vi "01AMT800_AnalyzeReceive.vi"(8 "error in (no error)":errorcluster, 10 "String":string, 11 "Enum":enum16{"Initialize", "Analyze"}(ring)) -> (0 "error out":errorcluster, 3 "Data":T1)   [LabVIEW 2015]
uses:
  <vilib>/regexp/Match Regular Expression.xnode
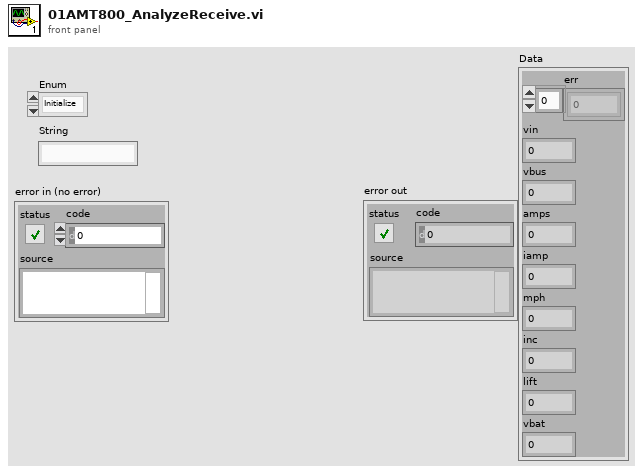
[diagram p1: front panel]
types:
  T1 = cluster{"err":i32[], "vin":i32, "vbus":i32, "amps":i32, "iamp":i32, "mph":i32, "inc":i32, "lift":i32, "vbat":i32}
  T2 = enum16{"Initialize", "Next", "Send RSET", "Set MPH", "Set INC", "Part to 0"}
  T3 = enum16{"Initialize", "FootReceive", "FootDisplay"}
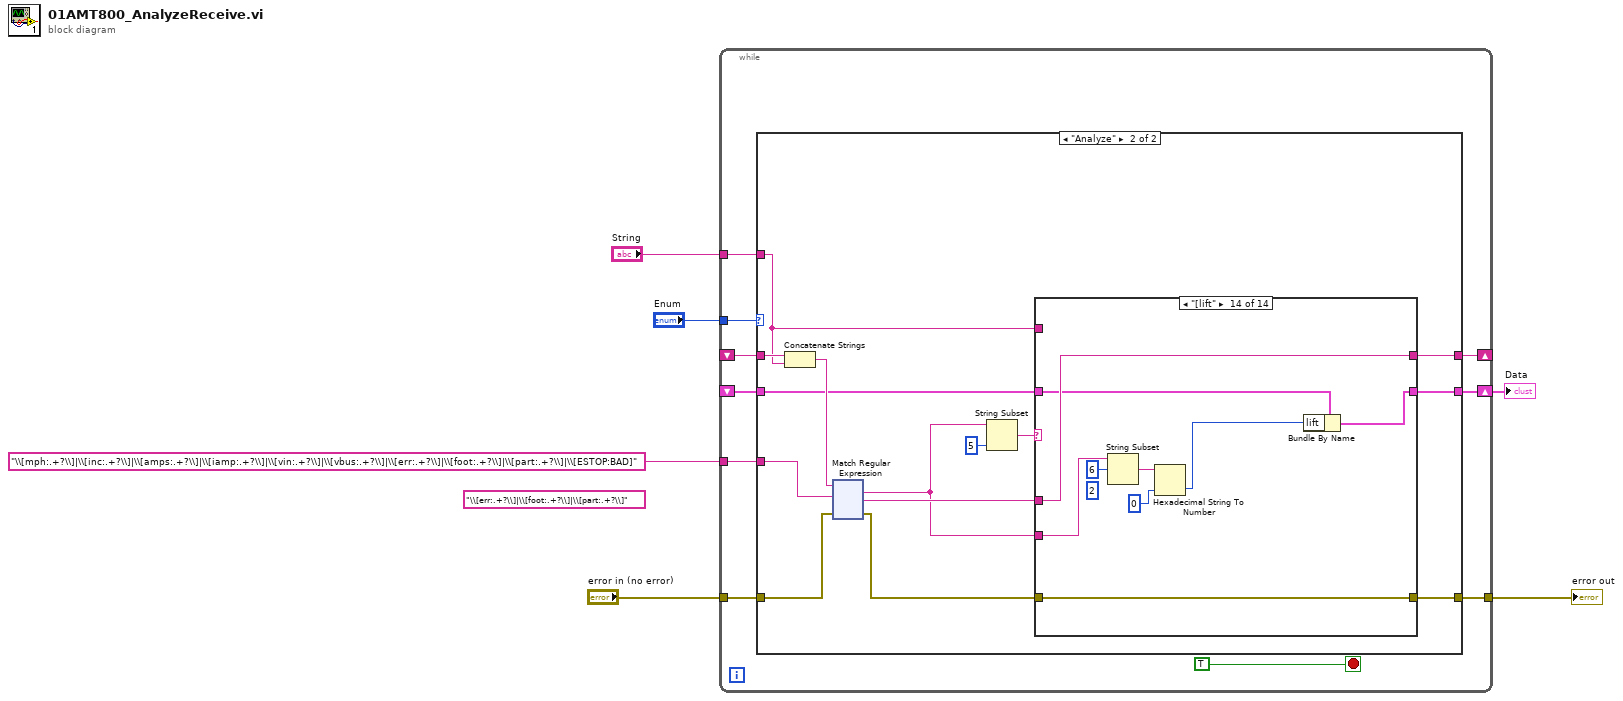
[diagram p0: block diagram]
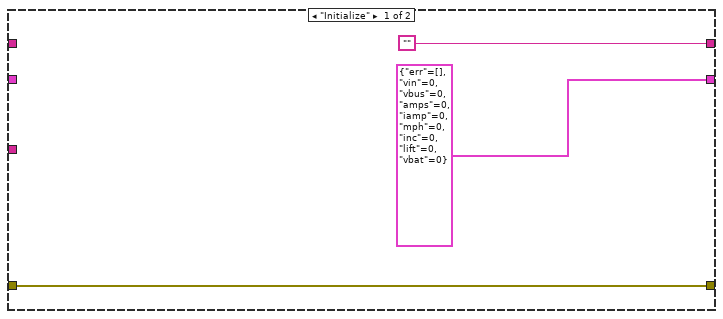
[diagram p2: hidden frame]
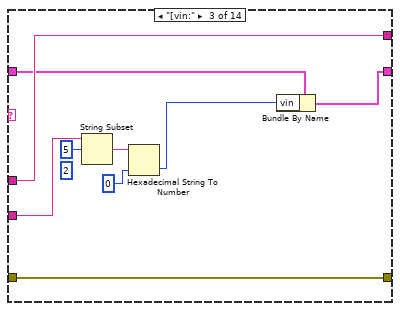
[diagram p5: hidden frame]
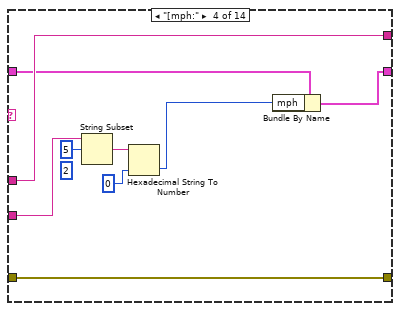
[diagram p6: hidden frame]
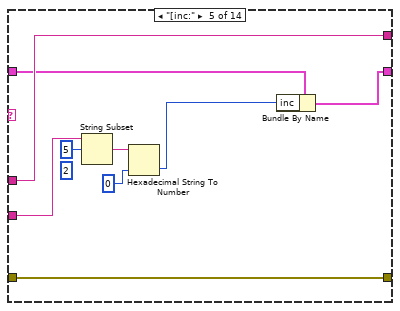
[diagram p7: hidden frame]
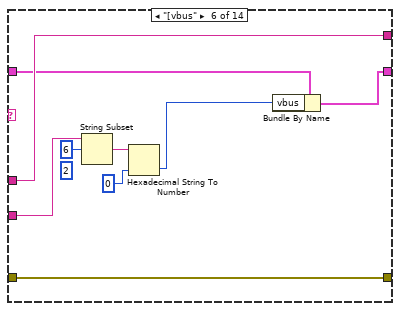
[diagram p8: hidden frame]
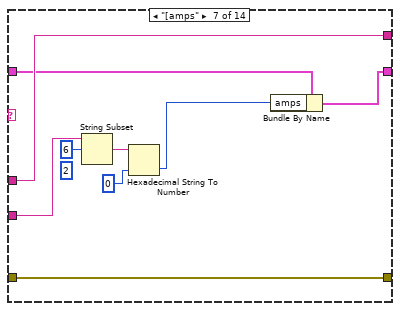
[diagram p9: hidden frame]
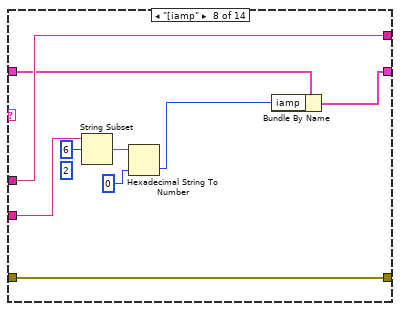
[diagram p10: hidden frame]
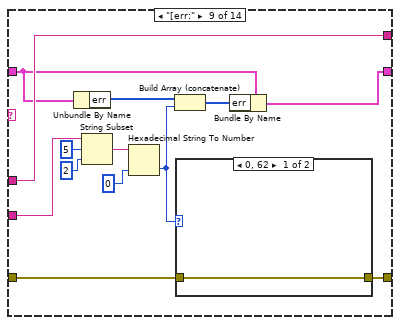
[diagram p11: hidden frame]
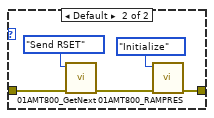
[diagram p12: hidden frame]
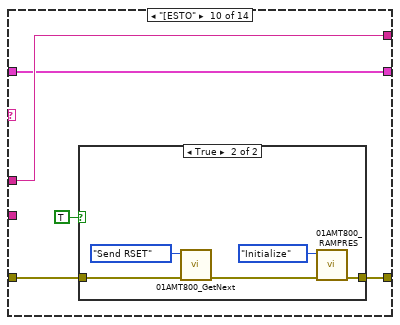
[diagram p13: hidden frame]
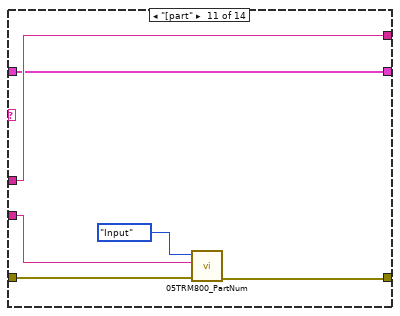
[diagram p15: hidden frame]
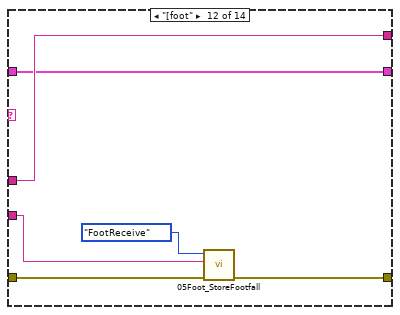
[diagram p16: hidden frame]
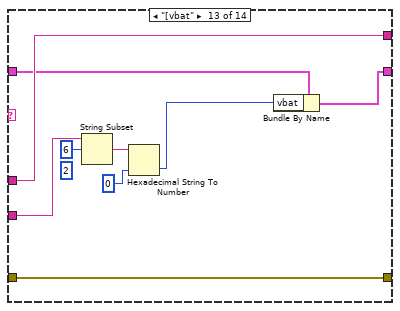
[diagram p17: hidden frame]
diagram:
  (unwired) "\\[err:.+?\\]|\\[foot:.+?\\]|\\[part:.+?\\]" ("regular expression")
  n1 = while {
    tunnel: "error in (no error)" -> [w13]
    tunnel: [w14] -> w5
    tunnel: "Enum" -> [w15]
    shift-right: [w12] -> _
    shift-left: _ -> [w11]
    tunnel: "String" -> [w10]
    tunnel: "\\[mph:.+?\\]|\\[inc:.+?\\]|\\[amps:.+?\\]|\\[iamp:.+?\\]|\\[vin:.+?\\]|\\[vbus:.+?\\]|\\[err:.+?\\]|\\[foot:.+?\\]|\\[part:.+?\\]|\\[ESTOP:BAD]" ("regular expression") -> [w9]
    shift-right: [w8] -> w1
    shift-left: _ -> [w7]
    stop <- TRUE stop-if-true
    n2 = case shown="\"Analyze\"" w15 {
      tunnel: [w19 w29] -> w14
      tunnel: w13 -> [w19 w26]
      tunnel: ["" w31] -> w12
      tunnel: w11 -> [_ w33]
      tunnel: w10 -> [_ w32]
      tunnel: w9 -> [_ w28]
      tunnel: [T1 {"err"=[], "vin"=0, "vbus"=0, "amps"=0, "iamp"=0, "mph"=0, "inc"=0, "lift"=0, "vbat"=0} w20] -> w8
      tunnel: w7 -> [_ w21]
      frame "Initialize" {
      }
      frame "Analyze" {
        n3 = Concatenate Strings(w33, w32) -> (w27:string)
        n4 = xnode "Match Regular Expression"("input string"=w27, "regular expression"=w28, "error in"=w26) -> ("whole match"=w22:string, "after match"=w30:string, "error out"=w25:errorcluster)  [unwired: 3 in, 2 out]
        n5 = String Subset(string=w22, length (rest)=5 ("length (rest)")) -> (substring=w24:string)  [unwired: 1 in]
        n6 = case shown="\"[lift\"" w24 {
          tunnel: w32 -> [w150 _ _ _ _ _ _ _ _ _ _ _ _ _]
          tunnel: [w150 w153 w162 w171 w180 w189 w198 w207 w220 w231 w243 w249 w258 w267] -> w31
          tunnel: w30 -> [_ w153 w162 w171 w180 w189 w198 w207 w220 w231 w243 w249 w258 w267]
          tunnel: [w149 w152 w154 w163 w172 w181 w190 w199 w210 w228 w241 w246 w250 w259] -> w29
          tunnel: w25 -> [w149 w152 w154 w163 w172 w181 w190 w199 w219 w230 w242 w247 w250 w259]
          tunnel: w22 -> [_ _ w158 w167 w176 w185 w194 w203 w215 _ w240 w245 w254 w263]
          tunnel: w21 -> [w148 w151 w157 w166 w175 w184 w193 w202 w212 w229 w238 w248 w253 w262]
          tunnel: [w148 w151 w156 w165 w174 w183 w192 w201 w211 w229 w238 w248 w252 w261] -> w20
          frame "" {
          }
          frame Default {
          }
          frame "[vin:" {
            (unwired) 2 ("length (rest)")
            n7 = String Subset(string=w158, offset (0)=5) -> (substring=w160:string)  [unwired: 1 in]
            n8 = Hexadecimal String To Number(string=w160, default (0uL)=0 ("default (0 U32)")) -> (number=w155:i32)  [unwired: 1 in, 1 out]
            n9 = Bundle By Name(cluster=w157, "vin"=w155) -> (w156:T1)
          }
          frame "[mph:" {
            (unwired) 2 ("length (rest)")
            n10 = String Subset(string=w167, offset (0)=5) -> (substring=w169:string)  [unwired: 1 in]
            n11 = Hexadecimal String To Number(string=w169, default (0uL)=0 ("default (0 U32)")) -> (number=w164:i32)  [unwired: 1 in, 1 out]
            n12 = Bundle By Name(cluster=w166, "mph"=w164) -> (w165:T1)
          }
          frame "[inc:" {
            (unwired) 2 ("length (rest)")
            n13 = String Subset(string=w176, offset (0)=5) -> (substring=w178:string)  [unwired: 1 in]
            n14 = Hexadecimal String To Number(string=w178, default (0uL)=0 ("default (0 U32)")) -> (number=w173:i32)  [unwired: 1 in, 1 out]
            n15 = Bundle By Name(cluster=w175, "inc"=w173) -> (w174:T1)
          }
          frame "[vbus" {
            (unwired) 2 ("length (rest)")
            n16 = String Subset(string=w185, offset (0)=6) -> (substring=w187:string)  [unwired: 1 in]
            n17 = Hexadecimal String To Number(string=w187, default (0uL)=0 ("default (0 U32)")) -> (number=w182:i32)  [unwired: 1 in, 1 out]
            n18 = Bundle By Name(cluster=w184, "vbus"=w182) -> (w183:T1)
          }
          frame "[amps" {
            (unwired) 2 ("length (rest)")
            n19 = String Subset(string=w194, offset (0)=6) -> (substring=w196:string)  [unwired: 1 in]
            n20 = Hexadecimal String To Number(string=w196, default (0uL)=0 ("default (0 U32)")) -> (number=w191:i32)  [unwired: 1 in, 1 out]
            n21 = Bundle By Name(cluster=w193, "amps"=w191) -> (w192:T1)
          }
          frame "[iamp" {
            (unwired) 2 ("length (rest)")
            n22 = String Subset(string=w203, offset (0)=6) -> (substring=w205:string)  [unwired: 1 in]
            n23 = Hexadecimal String To Number(string=w205, default (0uL)=0 ("default (0 U32)")) -> (number=w200:i32)  [unwired: 1 in, 1 out]
            n24 = Bundle By Name(cluster=w202, "iamp"=w200) -> (w201:T1)
          }
          frame "[err:" {
            n25 = Unbundle By Name(w212) -> ("err"=w214:i32[])
            n26 = String Subset(string=w215, offset (0)=5, length (rest)=2 ("length (rest)")) -> (substring=w216:string)
            n27 = Hexadecimal String To Number(string=w216, default (0uL)=0 ("default (0 U32)")) -> (number=w208:i32)  [unwired: 1 in, 1 out]
            n28 = Build Array (concatenate)(w214, w208) -> (w213:i32[])
            n29 = case shown="0, 62" w208 {
              tunnel: w219 -> [w221 w226]
              tunnel: [w221 w223] -> w210
              frame 0, 62 {
              }
              frame Default {
                n30 = call "01AMT800_GetNext.vi"("error in (no error)"=w226, "Enum"=T2."Send RSET") -> ("error out"=w224:errorcluster)  [unwired: 8 in, 1 out]
                n31 = call "01AMT800_RAMPRES.vi"("error in (no error)"=w224, "Enum"=enum16{"Initialize", "Set"}."Initialize") -> ("error out"=w223:errorcluster)  [unwired: 7 in, 2 out]
              }
            }
            n32 = Bundle By Name(cluster=w212, "err"=w213) -> (w211:T1)
          }
          frame "[ESTO" {
            n33 = case shown="True" TRUE {
              tunnel: w230 -> [w232 w237]
              tunnel: [w232 w233] -> w228
              frame False {
              }
              frame True {
                n34 = call "01AMT800_GetNext.vi"("error in (no error)"=w237, "Enum"=T2."Send RSET") -> ("error out"=w234:errorcluster)  [unwired: 8 in, 1 out]
                n35 = call "01AMT800_RAMPRES.vi"("error in (no error)"=w234, "Enum"=enum16{"Initialize", "Set"}."Initialize") -> ("error out"=w233:errorcluster)  [unwired: 7 in, 2 out]
              }
            }
          }
          frame "[part" {
            n36 = call "05TRM800_PartNum.vi"("error in (no error)"=w242, "Input"=w240, "Enum"=enum16{"Initialize", "Get", "Input"}."Input") -> ("error out"=w241:errorcluster)  [unwired: 7 in, 1 out]
          }
          frame "[foot" {
            n37 = call "05Foot_StoreFootfall.vi"("error in (no error)"=w247, "FootIn"=w245, "Enum"=T3."FootReceive") -> ("error out"=w246:errorcluster)  [unwired: 7 in, 1 out]
          }
          frame "[vbat" {
            (unwired) 2 ("length (rest)")
            n38 = String Subset(string=w254, offset (0)=6) -> (substring=w256:string)  [unwired: 1 in]
            n39 = Hexadecimal String To Number(string=w256, default (0uL)=0 ("default (0 U32)")) -> (number=w251:i32)  [unwired: 1 in, 1 out]
            n40 = Bundle By Name(cluster=w253, "vbat"=w251) -> (w252:T1)
          }
          frame "[lift" {
            (unwired) 2 ("length (rest)")
            n41 = String Subset(string=w263, offset (0)=6) -> (substring=w265:string)  [unwired: 1 in]
            n42 = Hexadecimal String To Number(string=w265, default (0uL)=0 ("default (0 U32)")) -> (number=w260:i32)  [unwired: 1 in, 1 out]
            n43 = Bundle By Name(cluster=w262, "lift"=w260) -> (w261:T1)
          }
        }
      }
    }
  }
  "error out" <- w5
  "Data" <- w1
